vi "Create RIO DAS Files.vi"(6 "Serial Numbers":string[](array[string]), 9 "Base Filepath":path, 10 "File Index In":i32) -> (0 "Bank2 Filepath":path, 1 "Bank1 Filepath":path, 2 "File Index Out":i32, 3 "Anomaly Filepath":path)   [LabVIEW 2018]
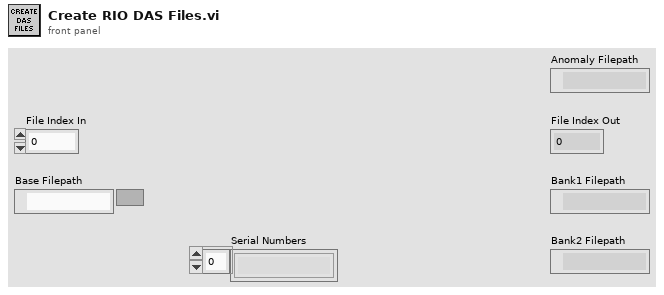
[diagram p1: front panel]
types:
  T1 = enum16{"open", "replace", "create", "open or create", "replace or create", "replace or create with confirmation"}
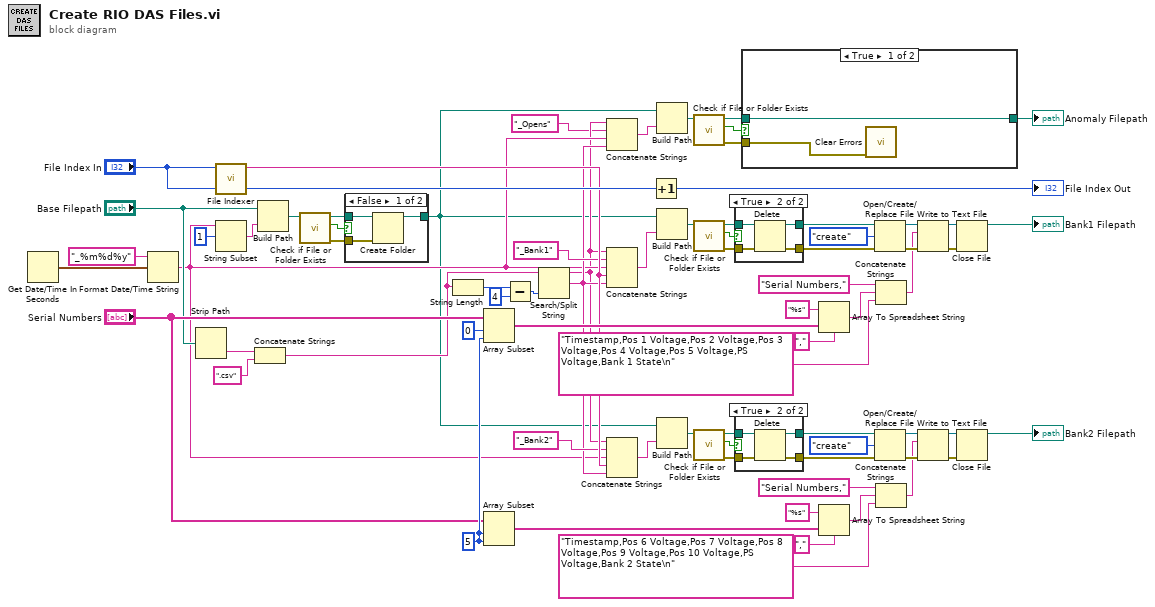
[diagram p0: block diagram]
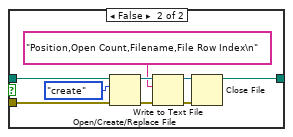
[diagram p3: hidden frame]
diagram:
  w39 = 5 ("length")
  n1 = Get Date/Time In Seconds() -> (seconds since 1Jan1904=w1:timestamp)
  n2 = Format Date/Time String(time format string (%c)="_%m%d%y", seconds (now)=w1) -> (date/time string=w14:string)  [unwired: 1 in]
  n3 = Strip Path(path="Base Filepath") -> (name=w48:string)  [unwired: 1 out]
  n4 = call "File Indexer.vi"("File Index In"="File Index In") -> ("File Indicator Out"=w20:string)  [unwired: 10 in]
  n5 = String Subset(string=w14, offset (0)=1) -> (substring=w50:string)  [unwired: 1 in]
  n6 = Concatenate Strings(w48, ".csv" ("string")) -> (w21:string)
  n7 = Build Path(base path="Base Filepath", name or relative path=w50) -> (appended path=w6:path)
  n8 = call <vilib>:"Check if File or Folder Exists.vi"("path"=w6) -> ("error out"=w2:errorcluster, "file or folder exists?"=w5:bool, "dup path"=w4:path)  [unwired: 8 in]
  n9 = case shown="False" w5 {
    tunnel: w4 -> [w77 w78]
    tunnel: [w76 w78] -> w3
    tunnel: w2 -> [w75 _]
    frame False {
      n10 = Create Folder(path (use dialog)=w77, error in=w75) -> (created path=w76:path)  [unwired: 1 in, 2 out]
    }
    frame True {
    }
  }
  n11 = String Length(string=w21) -> (length=w55:i32)
  n12 = Array Subset(array="Serial Numbers", index=0, length=w39) -> (w36:string[])
  n13 = Array Subset(array="Serial Numbers", index=w39, length=w39) -> (w37:string[])
  n14 = Subtract(x=w55, y=4) -> (x-y=w53:i32)
  n15 = Search/Split String(string=w21, offset (0)=w53) -> (substring before match=w12:string, match + rest of string=w15:string)  [unwired: 1 in, 1 out]
  n16 = Concatenate Strings(w12, "_Opens" ("string"), w14, w15) -> (w13:string)
  n17 = Concatenate Strings(w12, "_Bank1" ("string"), w14, w20, w15) -> (w51:string)
  n18 = Concatenate Strings(w12, "_Bank2" ("string"), w14, w20, w15) -> (w22:string)
  n19 = Increment(x="File Index In") -> (x+1=→"File Index Out":i32)
  n20 = Build Path(base path=w3, name or relative path=w13) -> (appended path=w16:path)
  n21 = Build Path(base path=w3, name or relative path=w51) -> (appended path=w58:path)
  n22 = Build Path(base path=w3, name or relative path=w22) -> (appended path=w34:path)
  n23 = call <vilib>:"Check if File or Folder Exists.vi"("path"=w16) -> ("error out"=w8:errorcluster, "file or folder exists?"=w7:bool, "dup path"=w9:path)  [unwired: 8 in]
  n24 = call <vilib>:"Check if File or Folder Exists.vi"("path"=w58) -> ("error out"=w72:errorcluster, "file or folder exists?"=w59:bool, "dup path"=w60:path)  [unwired: 8 in]
  n25 = call <vilib>:"Check if File or Folder Exists.vi"("path"=w34) -> ("error out"=w25:errorcluster, "file or folder exists?"=w33:bool, "dup path"=w32:path)  [unwired: 8 in]
  n26 = case shown="True" w59 {
    tunnel: w60 -> [w80 w84]
    tunnel: [w80 w83] -> w71
    tunnel: w72 -> [w79 w82]
    tunnel: [w79 w81] -> w73
    frame False {
    }
    frame True {
      n27 = Delete(path (use dialog)=w84, error in=w82) -> (deleted path=w83:path, error out=w81:errorcluster)  [unwired: 3 in, 1 out]
    }
  }
  n28 = case shown="True" w33 {
    tunnel: w32 -> [w86 w90]
    tunnel: [w86 w89] -> w26
    tunnel: w25 -> [w85 w88]
    tunnel: [w85 w87] -> w24
    frame False {
    }
    frame True {
      n29 = Delete(path (use dialog)=w90, error in=w88) -> (deleted path=w89:path, error out=w87:errorcluster)  [unwired: 3 in, 1 out]
    }
  }
  n30 = case shown="True" w7 {
    tunnel: w9 -> [w92 w97]
    tunnel: w8 -> [w91 w96]
    tunnel: [w92 w93] -> w10
    frame True {
      n31 = call <vilib>:"Clear Errors.vi"("error in (no error)"=w91) -> ()  [unwired: 5 in, 2 out]
    }
    frame False {
      n32 = Open/Create/Replace File(file path (use dialog)=w97, error in=w96, operation (0:open)=T1."create") -> (refnum out=w100:refnum<file>, error out=w98:errorcluster)  [unwired: 3 in, 1 out]
      n33 = Write to Text File(file (use dialog)=w100, text="Position,Open Count,Filename,File Row Index\n", error in=w98) -> (refnum out=w101:refnum<file>, error out=w99:errorcluster)  [unwired: 1 in, 1 out]
      n34 = Close File(refnum=w101, error in=w99) -> (path=w93:path)  [unwired: 1 out]
    }
  }
  "Anomaly Filepath" <- w10
  n35 = Array To Spreadsheet String(delimiter (Tab)=",", array=w36, 3:"%s" ("format string")) -> (spreadsheet string=w61:string)
  n36 = Array To Spreadsheet String(delimiter (Tab)=",", array=w37, 3:"%s" ("format string")) -> (spreadsheet string=w45:string)
  n37 = Open/Create/Replace File(file path (use dialog)=w71, error in=w73, operation (0:open)=T1."create") -> (refnum out=w67:refnum<file>, error out=w69:errorcluster)  [unwired: 3 in, 1 out]
  n38 = Open/Create/Replace File(file path (use dialog)=w26, error in=w24, operation (0:open)=T1."create") -> (refnum out=w30:refnum<file>, error out=w28:errorcluster)  [unwired: 3 in, 1 out]
  n39 = Concatenate Strings("Serial Numbers," ("string"), w61, "Timestamp,Pos 1 Voltage,Pos 2 Voltage,Pos 3 Voltage,Pos 4 Voltage,Pos 5 Voltage,PS Voltage,Bank 1 State\n") -> (w64:string)
  n40 = Concatenate Strings("Serial Numbers," ("string"), w45, "Timestamp,Pos 6 Voltage,Pos 7 Voltage,Pos 8 Voltage,Pos 9 Voltage,Pos 10 Voltage,PS Voltage,Bank 2 State\n") -> (w23:string)
  n41 = Write to Text File(file (use dialog)=w67, text=w64, error in=w69) -> (refnum out=w66:refnum<file>, error out=w68:errorcluster)  [unwired: 1 in, 1 out]
  n42 = Write to Text File(file (use dialog)=w30, text=w23, error in=w28) -> (refnum out=w31:refnum<file>, error out=w29:errorcluster)  [unwired: 1 in, 1 out]
  n43 = Close File(refnum=w66, error in=w68) -> (path=→"Bank1 Filepath":path)  [unwired: 1 out]
  n44 = Close File(refnum=w31, error in=w29) -> (path=→"Bank2 Filepath":path)  [unwired: 1 out]
